vi "GlobalVaribleDeclaration.vi"() -> ()   [LabVIEW 2019]
panel:
  in  "Age":dbl
  out "Is Pass or fail":bool
  in  "Your Full name":string
  in  "Your Marks":dbl
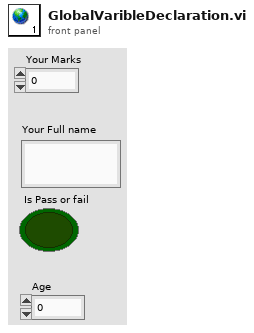
[diagram p1: front panel]
diagram:
